vi "Read Rank.vi"(8 "error in":errorcluster, 11 "SA Path Group in":refnum<class "SA 8GHz Path Group.lvclass">) -> (0 "error out":errorcluster, 2 "Rank":dbl, 3 "SA Path Group out":refnum<class "SA 8GHz Path Group.lvclass">)   [LabVIEW 2023, in "RFFixtureCharact.RMM.lvlib" / "SA 8GHz Path Group.lvclass"]
uses:
  SA 8GHz Path Group.lvclass
  SA 8GHz Path Group.lvclass/SA 8GHz Path Group.ctl
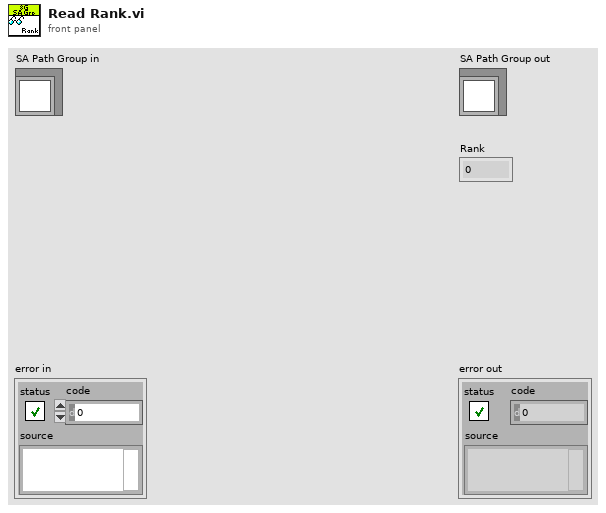
[diagram p1: front panel]
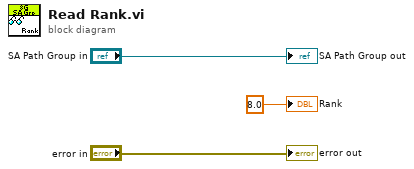
[diagram p0: block diagram]
diagram:
  "error out" <- "error in"
  "SA Path Group out" <- "SA Path Group in"
  "Rank" <- 8.0 ("Rank")
